vi "延时器.vi"(2 "当前值":dbl, 3 "dt":dbl=0.05, 4 "期望":dbl) -> (1 "输出":dbl)   [LabVIEW 2018]
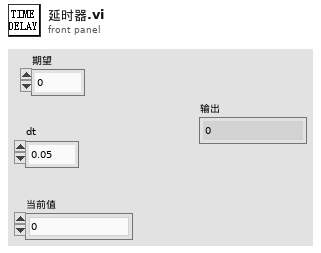
[diagram p1: front panel]
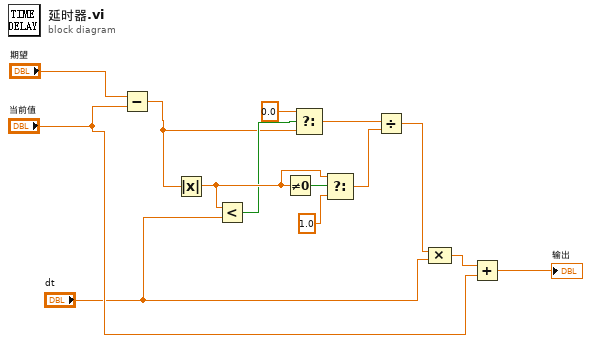
[diagram p0: block diagram]
diagram:
  n1 = Subtract(x="期望", y="当前值") -> (x-y=w2:dbl)
  n2 = Absolute Value(x=w2) -> (abs(x)=w6:dbl)
  n3 = Less?(x=w6, y="dt") -> (x < y?=w4:bool)
  n4 = Not Equal To 0?(x=w6) -> (x != 0?=w11:bool)
  n5 = Select(t=0.0, s=w4, f=w2) -> (s? t:f=w1:dbl)
  n6 = Select(t=w6, s=w11, f=1.0) -> (s? t:f=w13:dbl)
  n7 = Divide(x=w1, y=w13) -> (x/y=w14:dbl)
  n8 = Compound Arithmetic op=MULTIPLY(w14, "dt") -> (w10:dbl)
  n9 = Add(x=w10, y="当前值") -> (x+y=→"输出":dbl)
